vi "onlyVolumetric_Efficiency.vi"(0 "data":waveform(dbl)[](array[waveform])=[{"t0"=timestamp(3681324687.3726196 s since 1904-01-01), "dt"=0.1, "Y"=[21.99744063214368, 21.99744063214368, 21.99744063214368, 21.99744063214368], "attributes"=variant("NI_ChannelName"=variant(string "T_comp_in"), "NI_UnitDescription"=variant(string "Deg C"))}, {"t0"=timestamp(3681324687.3726196 s since 1904-01-01), "dt"=0.1, "Y"=[137.20192868203716, 137.20192868203716, 137.20192868203716, 137.20192868203716], "attributes"=variant("NI_ChannelName"=variant(string "T_comp_out"), "NI_UnitDescription"=variant(string "Deg C"))}, {"t0"=timestamp(3681324687.3726196 s since 1904-01-01), "dt"=0.1, "Y"=[105.8097492060228, 105.8097492060228, 105.8097492060228, 105.8097492060228], "attributes"=variant("NI_ChannelName"=variant(string "T_HEX_in"), "NI_UnitDescription"=variant(string "Deg C"))}, {"t0"=timestamp(3681324687.3726196 s since 1904-01-01), "dt"=0.1, "Y"=[27.607405549528632, 27.607405549528632, 27.607405549528632, 27.607405549528632], "attributes"=variant("NI_ChannelName"=variant(string "T_HEX_out"), "NI_UnitDescription"=variant(string "Deg C"))}, {"t0"=timestamp(3681324687.3726196 s since 1904-01-01), "dt"=0.1, "Y"=[2293.692067598917, 2293.692067598917, 2293.692067598917, 2293.692067598917], "attributes"=variant("NI_ChannelName"=variant(string "T_idler_t"), "NI_UnitDescription"=variant(string "Deg C"))}, {"t0"=timestamp(3681324687.3726196 s since 1904-01-01), "dt"=0.1, "Y"=[47.359214211488585, 47.359214211488585, 47.359214211488585, 47.359214211488585], "attributes"=variant("NI_ChannelName"=variant(string "T_idler_br"), "NI_UnitDescription"=variant(string "Deg C"))}, {"t0"=timestamp(3681324687.3726196 s since 1904-01-01), "dt"=0.1, "Y"=[63.14379772547072, 63.14379772547072, 63.14379772547072, 63.14379772547072], "attributes"=variant("NI_ChannelName"=variant(string "T_idler_bl"), "NI_UnitDescription"=variant(string "Deg C"))}, {"t0"=timestamp(3681324687.3726196 s since 1904-01-01), "dt"=0.1, "Y"=[37.48998084625662, 37.48998084625662, 37.48998084625662, 37.48998084625662], "attributes"=variant("NI_ChannelName"=variant(string "T_exp_surf"), "NI_UnitDescription"=variant(string "Deg C"))}, {"t0"=timestamp(3681324687.3726196 s since 1904-01-01), "dt"=0.1, "Y"=[2293.692067598917, 2293.692067598917, 2293.692067598917, 2293.692067598917], "attributes"=variant("NI_ChannelName"=variant(string "108"), "NI_UnitDescription"=variant(string "Deg C"))}, {"t0"=timestamp(3681324687.3726196 s since 1904-01-01), "dt"=0.1, "Y"=[2293.692067598917, 2293.692067598917, 2293.692067598917, 2293.692067598917], "attributes"=variant("NI_ChannelName"=variant(string "109"), "NI_UnitDescription"=variant(string "Deg C"))}, {"t0"=timestamp(3681324687.3726196 s since 1904-01-01), "dt"=0.1, "Y"=[2293.692067598917, 2293.692067598917, 2293.692067598917, 2293.692067598917], "attributes"=variant("NI_ChannelName"=variant(string "110"), "NI_UnitDescription"=variant(string "Deg C"))}, {"t0"=timestamp(3681324687.3726196 s since 1904-01-01), "dt"=0.1, "Y"=[2293.692067598917, 2293.692067598917, 2293.692067598917, 2293.692067598917], "attributes"=variant("NI_ChannelName"=variant(string "111"), "NI_UnitDescription"=variant(string "Deg C"))}, {"t0"=timestamp(3681324687.3726196 s since 1904-01-01), "dt"=0.1, "Y"=[2293.692067598917, 2293.692067598917, 2293.692067598917, 2293.692067598917], "attributes"=variant("NI_ChannelName"=variant(string "112"), "NI_UnitDescription"=variant(string "Deg C"))}, {"t0"=timestamp(3681324687.3726196 s since 1904-01-01), "dt"=0.1, "Y"=[2293.692067598917, 2293.692067598917, 2293.692067598917, 2293.692067598917], "attributes"=variant("NI_ChannelName"=variant(string "113"), "NI_UnitDescription"=variant(string "Deg C"))}, {"t0"=timestamp(3681324687.3726196 s since 1904-01-01), "dt"=0.1, "Y"=[2293.692067598917, 2293.692067598917, 2293.692067598917, 2293.692067598917], "attributes"=variant("NI_ChannelName"=variant(string "114"), "NI_UnitDescription"=variant(string "Deg C"))}, {"t0"=timestamp(3681324687.3726196 s since 1904-01-01), "dt"=0.1, "Y"=[2293.692067598917, 2293.692067598917, 2293.692067598917, 2293.692067598917], "attributes"=variant("NI_ChannelName"=variant(string "115"), "NI_UnitDescription"=variant(string "Deg C"))}, {"t0"=timestamp(3681324687.3726196 s since 1904-01-01), "dt"=0.1, "Y"=[6.24549875288, 5.86351236368, 6.43649194748, 5.0995395852800005], "attributes"=variant("NI_ChannelName"=variant(string "V_dot_exp_3000"))}, {"t0"=timestamp(3681324687.3726196 s since 1904-01-01), "dt"=0.1, "Y"=[1.1554134350520002, 1.1743768069680003, 1.1459317490940002, 1.1554134350520002], "attributes"=variant("NI_ChannelName"=variant(string "Tq_comp"))}, {"t0"=timestamp(3681324687.3726196 s since 1904-01-01), "dt"=0.1, "Y"=[49.0088736, 9.746512, -5.0406112000000025, 47.989072], "attributes"=variant("NI_ChannelName"=variant(string "N_comp"))}, {"t0"=timestamp(3681324687.3726196 s since 1904-01-01), "dt"=0.1, "Y"=[12.103964176338803, 12.048590187959302, 12.064411327496302, 12.096053606570303], "attributes"=variant("NI_ChannelName"=variant(string "P_comp_in"))}, {"t0"=timestamp(3681324687.3726196 s since 1904-01-01), "dt"=0.1, "Y"=[12.166878140449498, 12.1064238072918, 12.189150789507599, 12.1414236843831], "attributes"=variant("NI_ChannelName"=variant(string "P_comp_out"))}, {"t0"=timestamp(3681324687.3726196 s since 1904-01-01), "dt"=0.1, "Y"=[0.19104224250000007, 0.16503048750000007, 0.15320696250000007, 0.12483050250000005], "attributes"=variant("NI_ChannelName"=variant(string "Current"))}, {"t0"=timestamp(3681324687.3726196 s since 1904-01-01), "dt"=0.1, "Y"=[374.0384878, 371.9836168, 372.4103977, 372.9162121], "attributes"=variant("NI_ChannelName"=variant(string "Voltage_480"))}, {"t0"=timestamp(3681324687.3726196 s since 1904-01-01), "dt"=0.1, "Y"=[0.36160326047999997, 0.42537884015999994, 0.42537884015999994, -0.021050217600000032], "attributes"=variant("NI_ChannelName"=variant(string "V_dot_exp_1000"))}], 1 "Working Fluid":string="R134A.FLD", 2 "?":path=path "C:/Users/ASITest/Desktop/REFPROP", 4 "Comp Pressure In (PSI)":i32=18, 5 "Suction Volume":dbl=0.001803, 7 "Override Speed Entry?":i32=1, 9 "m_dot_wf":i32=21, 10 "Comp Temp In (C)":i32, 11 "error in (no error)":errorcluster, 12 "Speed (RPM)":i32, 13 "Comp Pressure Out (PSI)":i32=19, 14 "Override (RPM)":dbl=2000.0) -> (3 "Eff.":waveform(dbl)[](graph)=[{"t0"=timestamp(3693583526.984508 s since 1904-01-01), "dt"=0.01, "Y"=[0.0006711177998339175]}], 6 "V_eff":dbl=0.0006711177998339175, 15 "error out":errorcluster)   [LabVIEW 2016]
doc: "Select the file location where REFPROP can be called from on local disk & input to Front Panel.\n\nie. C:\\Users\\ASITest\\Desktop\\REFPROP\n\nDo not reference REFPROP in the shared drive but instead save the entire folder locally and reference it from there.\n\nREFPROP folder to be copied can be found here: \nS:\\101 - Engineering\\16 - Training\\2 - LabVIEW\\REFPROP\n\nThe two sub vi's that this vi depends on can be found here:\n\n S:\\009 - Testing\\02 - Performance Testing\\8 - Labview Sub VI\\REFPROP\\Any_Ref_enthalpy_funct_TP_REFPROP10.vi\n\n S:\\009 - Testing\\02 - Performance Testing\\8 - Labview Sub VI\\REFPROP\\Any_Ref_enthalpy_funct_PS_REFPROP10.vi\n\nThe two Any_Ref_enthalpy_funct_XX_REFPROP10 sub vi's need to be referenced and stored as two seperate files with in the same folder that is input on the front panel.\nThe _PS_ file depends on the results of the _TP_ file, and in order to ensure that they each are able to make independent computations at the same time, they need to be seperate files that are hard coded to their specific functions."
uses:
  <vilib>/Utility/error.llb/DialogType.ctl
panel:
  out "delta_Enthalpy":dbl=0.04096011811162725
  out "Ideal Enthalpy":dbl=421.12006460178327
  out "Eff.":waveform(dbl)[](array[waveform])=[{"t0"=timestamp(3681324687.3726196 s since 1904-01-01), "dt"=0.1, "Y"=[1.030568661423571]}]
  out "N [rev/s]":dbl=33.333333333333336
  out "m_dot":dbl=0.00014694807499999936
  out "Density_in":dbl=3.643264244813777
  out "Entropy_in":dbl=1.9024232360659565
  out "Enthalpy_in":dbl=421.07910448367164
  # "Point to where REFPROP is..."
  # "INPUT NEEDED"
  # "0 = N\n1 = Y"
  # "Data Index of Calc Characteristics"
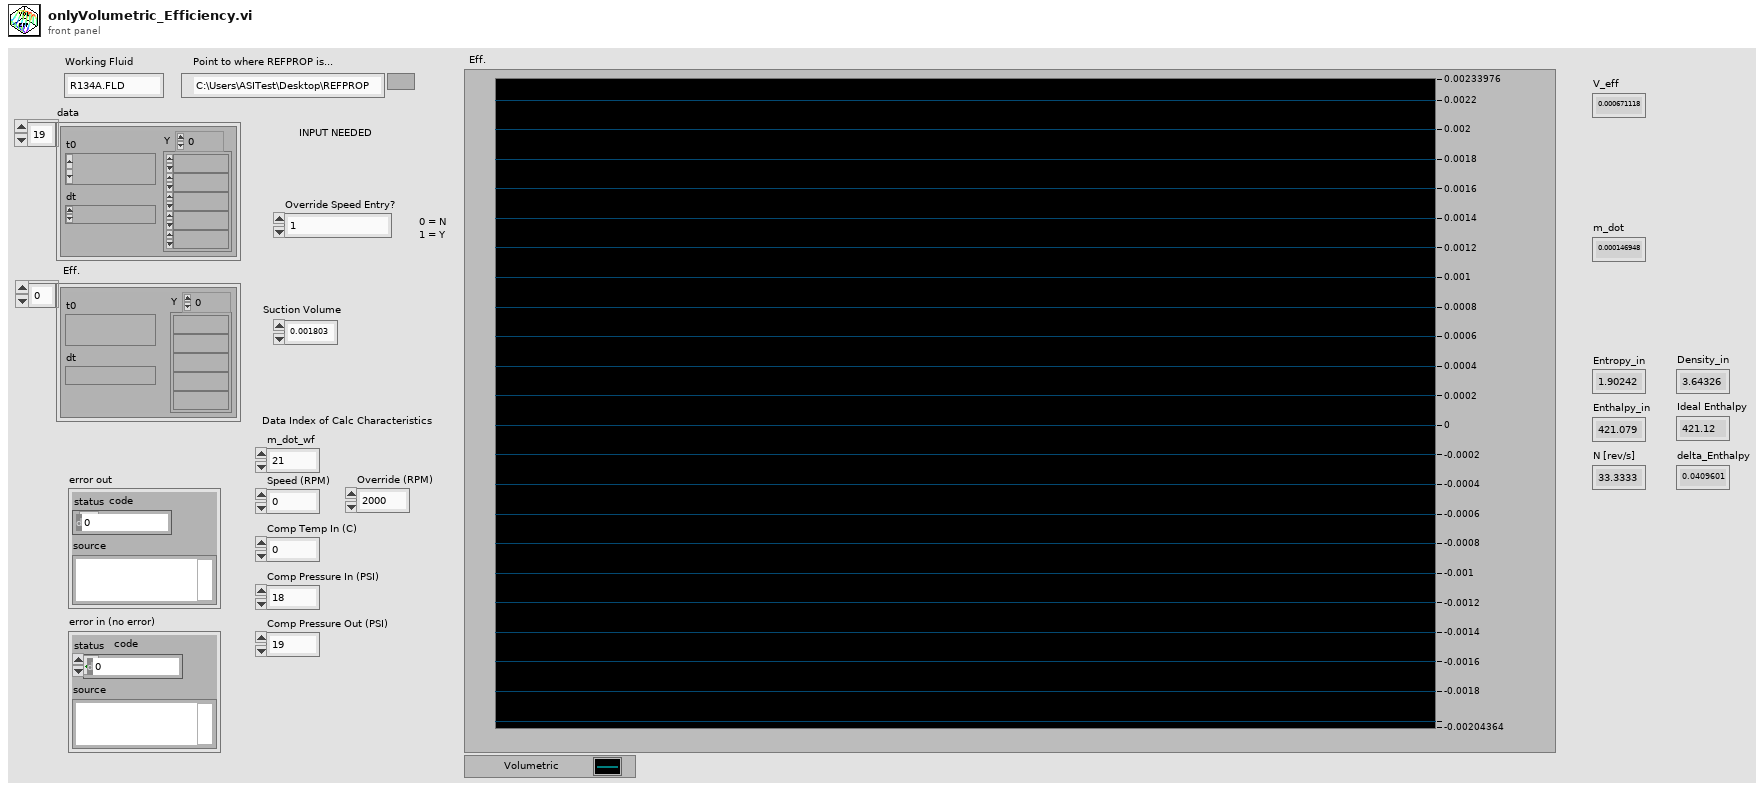
[diagram p1: front panel]
types:
  T1 = typedef "DialogType.ctl" = u16
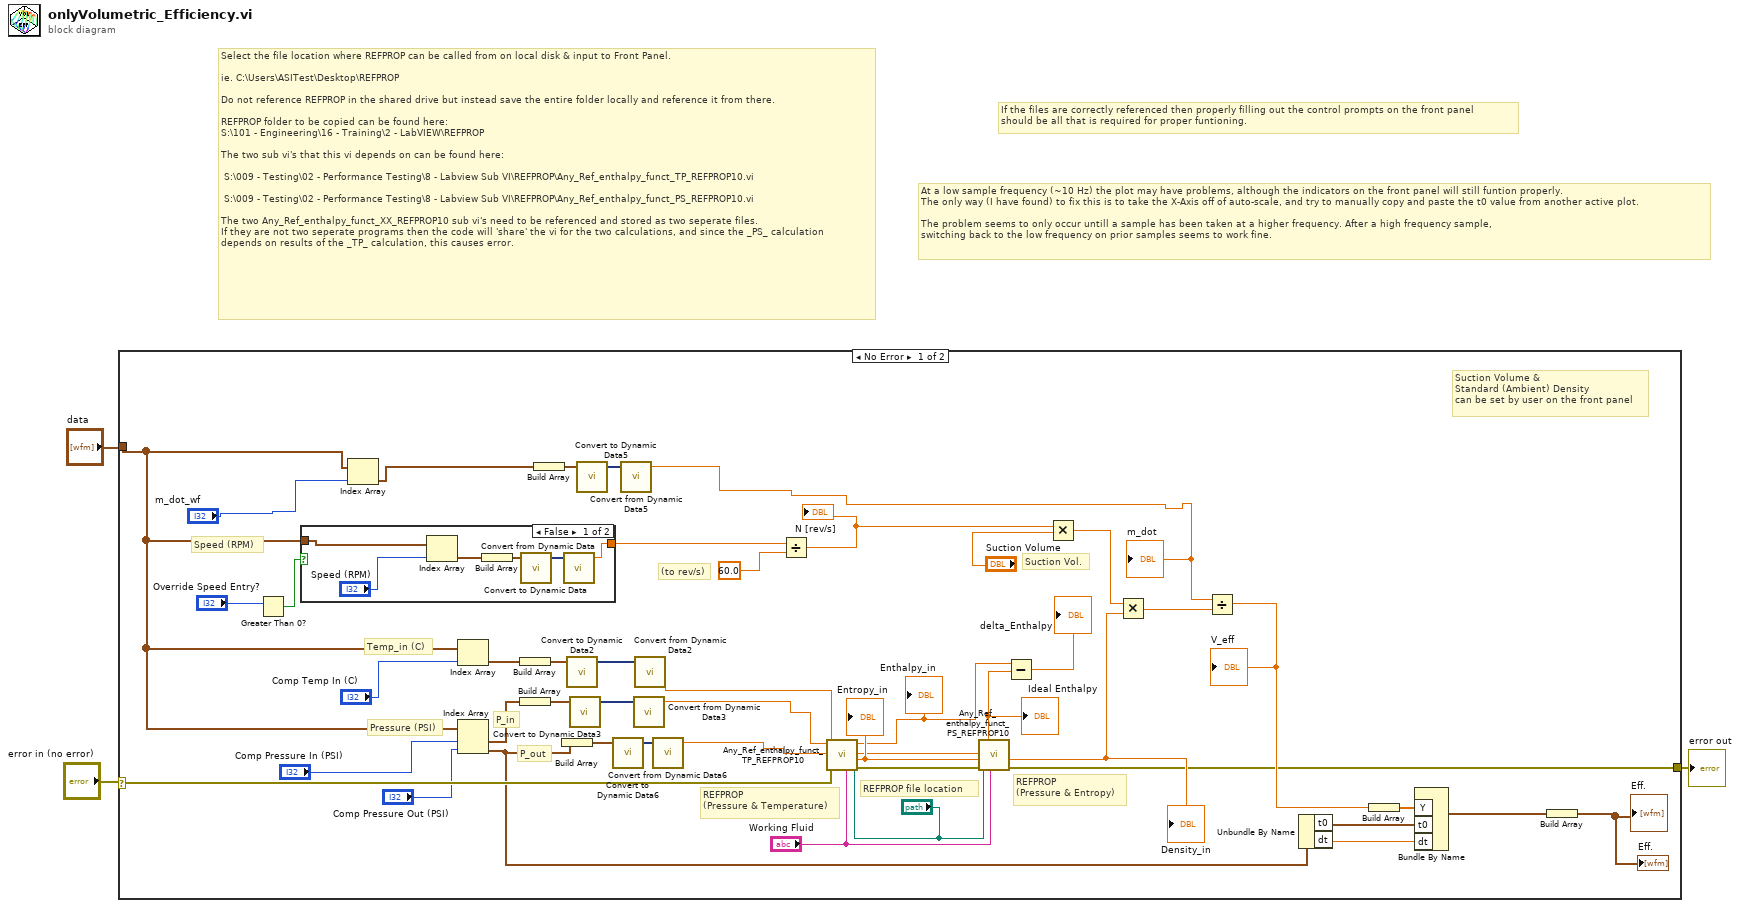
[diagram p0: block diagram]
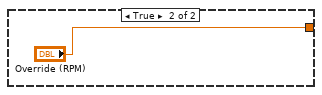
[diagram p2: hidden frame]
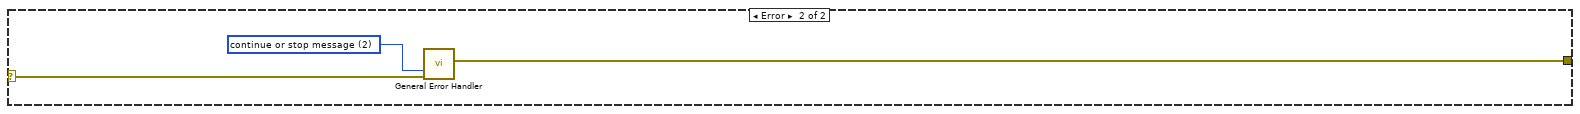
[diagram p3: hidden frame]
diagram:
  # "At a low sample frequency (~10 Hz) the plot may have problems, although the indicators on the front panel will still funtion properly.\nThe only way (I have found) to fix this is to take the X-Axis off of auto-scale, and try to manually copy and paste the t0 value from another active plot. \n\nThe problem seems to only occur untill a sample has been taken at a higher frequency. After a high frequency sample, \nswitching back to the low frequency on prior samples seems to work fine."
  # "If the files are correctly referenced then properly filling out the control prompts on the front panel \nshould be all that is required for proper funtioning."
  # "Select the file location where REFPROP can be called from on local disk & input to Front Panel.\n\nie. C:\\Users\\ASITest\\Desktop\\REFPROP\n\nDo not reference REFPROP in the shared drive but instead save the entire folder locally and reference it from there.\n\nREFPROP folder to be copied can be found here: \nS:\\101 - Engineering\\16 - Training\\2 - LabVIEW\\REFPROP\n\nThe two sub vi's that this vi depends on can be found here:\n\n S:\\009 - Testing\\02 - Performance Testing\\8 - Labview Sub VI\\REFPROP\\Any_Ref_enthalpy_funct_TP_REFPROP10.vi\n\n S:\\009 - Testing\\02 - Performance Testing\\8 - Labview Sub VI\\REFPROP\\Any_Ref_enthalpy_funct_PS_REFPROP10.vi\n\nThe two Any_Ref_enthalpy_funct_XX_REFPROP10 sub vi's need to be referenced and stored as two seperate files. \nIf they are not two seperate programs then the code will 'share' the vi for the two calculations, and since the _PS_ calculation\ndepends on results of the _TP_ calculation, this causes error."
  n1 = case shown="No Error" "error in (no error)" {
    selector: "error in (no error)" -> [w29 w56]
    tunnel: "data" -> [w9 _]
    tunnel: [w26 w57] -> w1
    frame No Error {
      # "Suction Vol."
      # "Suction Volume &\nStandard (Ambient) Density\ncan be set by user on the front panel"
      # "(to rev/s)"
      # "REFPROP\n(Pressure & Temperature)"
      # "REFPROP\n(Pressure & Entropy)"
      # "REFPROP file location"
      # "P_in"
      # "P_out"
      # "Pressure (PSI)"
      # "Temp_in (C)"
      # "Speed (RPM)"
      n2 = Greater Than 0?(x="Override Speed Entry?") -> (x > 0?=w10:bool)
      n3 = case shown="False" w10 {
        tunnel: [w49 "Override (RPM)"] -> w45
        tunnel: w9 -> [w51 _]
        frame False {
          n4 = Index Array(array=w51, index="Speed (RPM)") -> (element=w53:waveform(dbl))
          n5 = Build Array(w53) -> (w54:waveform(dbl)[])
          n6 = call "Convert to Dynamic Data"("Array of Waveforms"=w54) -> ("Dynamic Data Type"=w50:dynamicdata)  [unwired: 3 in]
          n7 = call "Convert from Dynamic Data"("Dynamic Data Type"=w50, "Channel"=w50) -> ("Scalar"=w49:dbl)  [unwired: 2 in]
        }
        frame True {
        }
      }
      n8 = Index Array(array=w9, index="m_dot_wf") -> (element=w7:waveform(dbl))
      n9 = Index Array(array=w9, index="Comp Temp In (C)") -> (element=w36:waveform(dbl))
      n10 = Index Array(array=w9, index #1="Comp Pressure In (PSI)", index #2="Comp Pressure Out (PSI)") -> (element #1=w33:waveform(dbl), element #2=w15:waveform(dbl))
      n11 = Build Array(w36) -> (w40:waveform(dbl)[])
      n12 = Build Array(w33) -> (w37:waveform(dbl)[])
      n13 = Build Array(w7) -> (w47:waveform(dbl)[])
      n14 = Build Array(w15) -> (w31:waveform(dbl)[])
      n15 = call "Convert to Dynamic Data2"("Array of Waveforms"=w40) -> ("Dynamic Data Type"=w41:dynamicdata)  [unwired: 3 in]
      n16 = call "Convert to Dynamic Data3"("Array of Waveforms"=w37) -> ("Dynamic Data Type"=w38:dynamicdata)  [unwired: 3 in]
      n17 = call "Convert to Dynamic Data5"("Array of Waveforms"=w47) -> ("Dynamic Data Type"=w48:dynamicdata)  [unwired: 3 in]
      n18 = call "Convert to Dynamic Data6"("Array of Waveforms"=w31) -> ("Dynamic Data Type"=w32:dynamicdata)  [unwired: 3 in]
      n19 = call "Convert from Dynamic Data5"("Dynamic Data Type"=w48) -> ("Scalar"=w6:dbl)  [unwired: 3 in]
      "m_dot" <- w6
      n20 = call "Convert from Dynamic Data3"("Dynamic Data Type"=w38) -> ("Scalar"=w5:dbl)  [unwired: 3 in]
      n21 = call "Convert from Dynamic Data2"("Dynamic Data Type"=w41) -> ("Scalar"=w39:dbl)  [unwired: 3 in]
      n22 = call "Convert from Dynamic Data6"("Dynamic Data Type"=w32) -> ("Scalar"=w4:dbl)  [unwired: 3 in]
      n23 = Divide(x=w45, y=60.0) -> (x/y=w34:dbl)
      "N [rev/s]" <- w34
      n24 = call "Any_Ref_enthalpy_funct_TP_REFPROP10.vi"("Input Temperature [C]"=w39, "Input Pressure [kPa]"=w5, "error in (no error)"=w29, 4:"?", "Fluidofinterest"="Working Fluid") -> ("Enthalpy [kJ/kg]"=w22:dbl, "Entropy"=w28:dbl, "Density"=w43:dbl, "error out"=w27:errorcluster)  [unwired: 2 in]
      "Enthalpy_in" <- w22
      "Entropy_in" <- w28
      "Density_in" <- w43
      n25 = call "Any_Ref_enthalpy_funct_PS_REFPROP10.vi"("Pressure Out (kPa)"=w4, "S_in"=w28, "error in (no error)"=w27, "Fluidofinterest"="Working Fluid", 5:"?") -> ("h2_s"=w23:dbl, "error out"=w26:errorcluster)  [unwired: 4 in]
      "Ideal Enthalpy" <- w23
      n26 = Subtract(x=w23, y=w22) -> (x-y=→"delta_Enthalpy":dbl)
      n27 = Multiply(x="Suction Volume", y=w34) -> (x*y=w44:dbl)
      n28 = Multiply(x=w44, y=w43) -> (x*y=w42:dbl)
      n29 = Divide(x=w6, y=w42) -> (x/y=w35:dbl)
      "V_eff" <- w35
      n30 = Unbundle By Name(w15) -> ("t0"=w17:timestamp, "dt"=w18:dbl)
      n31 = Build Array(w35) -> (w16:dbl[])
      n32 = Bundle By Name ("Build Waveform")("Y"=w16, "t0"=w17, "dt"=w18) -> (w24:waveform(dbl))  [unwired: 1 in]
      n33 = Build Array(w24) -> (→"Eff." →"Eff.":waveform(dbl)[])
    }
    frame Error {
      w58 = T1 2 items=["no dialog", "OK message", "continue or stop message", "OK message + warnings", "continue/stop + warnings"] ("type of dialog (OK msg:1)")
      n34 = call <vilib>:"General Error Handler.vi"("type of dialog (OK msg:1)"=w58, "error in (no error)"=w56) -> ("error out"=w57:errorcluster)  [unwired: 9 in, 4 out]
    }
  }
  "error out" <- w1
